vi "Decode Binary Stream Part 2.vi"(11 "Bit Stream":bool[](array[boolean])) -> (2 "Packets Out":T1[](array[typedef]), 3 "Bit Stream Out":bool[](array[boolean]))   [LabVIEW 2019, in "Day 16.lvlib"]
uses:
  Day 16.lvlib
  Controls/Packet.ctl
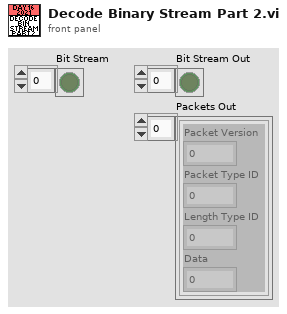
[diagram p1: front panel]
types:
  T1 = typedef "Day 16.lvlib/Packet.ctl" = cluster{"Packet Version":u32, "Packet Type ID":u32, "Length Type ID":u32, "Data":u64}
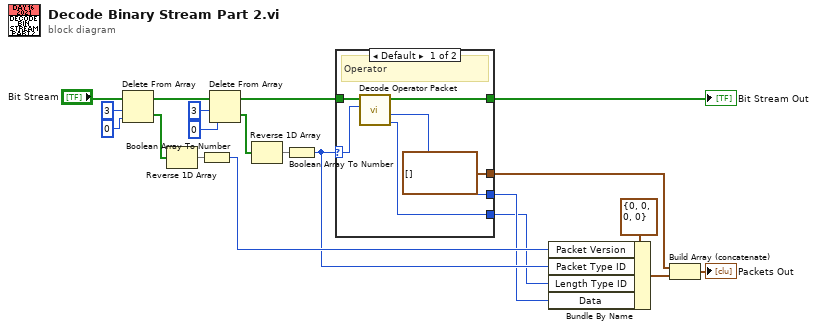
[diagram p0: block diagram]
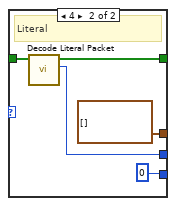
[diagram p2: hidden frame]
diagram:
  n1 = Delete From Array(array="Bit Stream", length=3, index=0) -> (deleted portion=w15:bool[], array with subset deleted=w17:bool[])
  n2 = Reverse 1D Array(array=w15) -> (reversed array=w14:bool[])
  n3 = Boolean Array To Number(Boolean array=w14) -> (number=w10:u32)
  n4 = Delete From Array(array=w17, length=3, index=0) -> (deleted portion=w12:bool[], array with subset deleted=w7:bool[])
  n5 = Reverse 1D Array(array=w12) -> (reversed array=w13:bool[])
  n6 = Boolean Array To Number(Boolean array=w13) -> (number=w9:u32)
  n7 = case shown="Default" w9 {
    selector: w9 -> [w22 _]
    tunnel: w7 -> [w26 w31]
    tunnel: [w25 w28] -> w2
    tunnel: [w24 w30] -> w6
    tunnel: [w23 u64 0 ("Length Type ID")] -> w5
    tunnel: [T1[] [] ("Packets Out") T1[] [] ("Packets Out")] -> w1
    frame Default {
      # "Operator"
      n8 = call "Decode Operator Packet.vi"("Type ID"=w22, "Bit Stream in"=w26) -> ("Length Type ID"=w23:u32, "Value"=w24:u64, "Bit Stream out"=w25:bool[])  [unwired: 6 in, 1 out]
    }
    frame 4 {
      # "Literal"
      n9 = call "Decode Literal Packet.vi"("Bit Stream In"=w31) -> ("Data"=w30:u64, "Bit Stream Out"=w28:bool[])  [unwired: 9 in]
    }
  }
  "Bit Stream Out" <- w2
  n10 = Bundle By Name(cluster=T1 {"Packet Version"=0, "Packet Type ID"=0, "Length Type ID"=0, "Data"=0} ("Packet"), "Packet Version"=w10, "Packet Type ID"=w9, "Length Type ID"=w5, "Data"=w6) -> (w8:T1)
  n11 = Build Array (concatenate)(w1, w8) -> (→"Packets Out":T1[])
